vi "PM100D_SetRngIndex.vi"(1 "PM16":bool, 5 "VISAin":refnum<visa-resource-name>, 7 "Unit":string, 9 "AUTO":bool, 11 "error in":errorcluster, 12 "SensType":i32, 13 "Rng_Array":string[](array[string]), 14 "Index":i32) -> (4 "VISAout":refnum<visa-resource-name>, 6 "lblRange":string, 8 "Numeric 2":dbl, 10 "AUTO?":bool, 15 "error out 2":errorcluster)   [LabVIEW 2011]
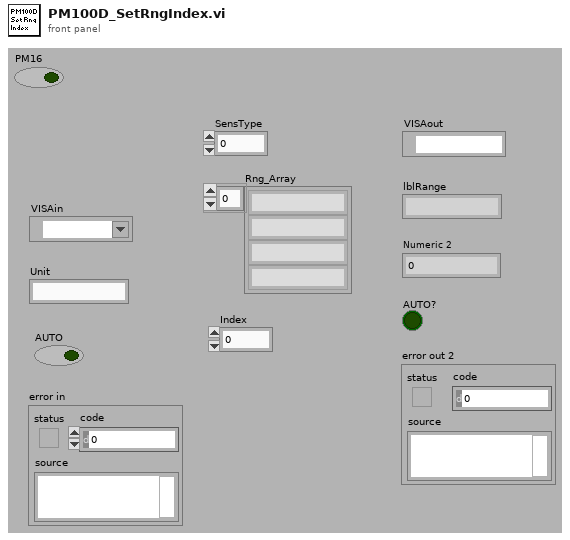
[diagram p1: front panel]
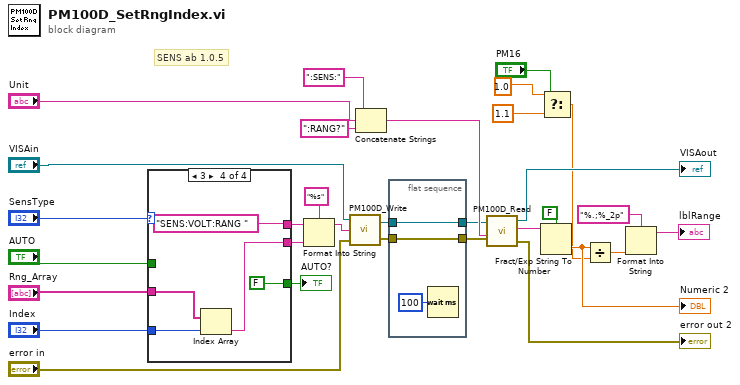
[diagram p0: block diagram]
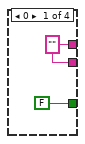
[diagram p2: hidden frame]
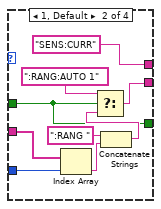
[diagram p3: hidden frame]
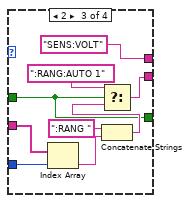
[diagram p4: hidden frame]
diagram:
  # "SENS ab 1.0.5"
  n1 = case shown="3" "SensType" {
    tunnel: [w33 "SENS:CURR" "SENS:VOLT" "SENS:VOLT:RANG " ("string")] -> w18
    tunnel: "Index" -> [_ w42 w51 w56]
    tunnel: "AUTO" -> [_ w34 w43 _]
    tunnel: [w33 w40 w49 w55] -> w20
    tunnel: "Rng_Array" -> [_ w39 w48 w54]
    tunnel: [FALSE ("AUTO") w34 w43 FALSE ("AUTO")] -> w28
    frame 0 {
      w33 = ""
    }
    frame 1, Default {
      n2 = Index Array(array=w39, index=w42) -> (element=w38:string)
      n3 = Concatenate Strings(":RANG " ("string"), w38) -> (w36:string)
      n4 = Select(t=":RANG:AUTO 1", s=w34, f=w36) -> (s? t:f=w40:string)
    }
    frame 2 {
      n5 = Index Array(array=w48, index=w51) -> (element=w45:string)
      n6 = Concatenate Strings(":RANG " ("string"), w45) -> (w44:string)
      n7 = Select(t=":RANG:AUTO 1", s=w43, f=w44) -> (s? t:f=w49:string)
    }
    frame 3 {
      n8 = Index Array(array=w54, index=w56) -> (element=w55:string)
    }
  }
  "AUTO?" <- w28
  n9 = Format Into String(format string="%s", initial string=w18, w20) -> (resulting string=w17:string)  [unwired: 1 in, 1 out]
  n10 = call "PM100D_Write.vi"("error in (no error)"="error in", "Command"=w17, "VISA in"="VISAin") -> ("error out"=w6:errorcluster, "VISA out"=w8:refnum<visa-resource-name>)
  n11 = Concatenate Strings(":SENS:" ("string"), "Unit", ":RANG?" ("string")) -> (w21:string)
  n12 = flat-sequence {
    tunnel: [w59] -> w7
    tunnel: w8 -> [w59]
    tunnel: w6 -> [w58]
    tunnel: [w58] -> w5
    frame #0 {
      n13 = Wait (ms)(milliseconds to wait=u32 100) -> ()  [unwired: 1 out]
    }
  }
  n14 = call "PM100D_Read.vi"("error in (no error)"=w5, "Command"=w21, "VISA in"=w7) -> ("error out"=→"error out 2":errorcluster, "ReadValue"=w12:string, "VISA out"=→"VISAout":refnum<visa-resource-name>)  [unwired: 1 in]
  n15 = Fract/Exp String To Number(use system decimal point (T)=FALSE, string=w12) -> (number=w14:dbl)  [unwired: 2 in, 1 out]
  "Numeric 2" <- w14
  n16 = Select(t=1.0 ("y"), s="PM16", f=1.1) -> (s? t:f=w3:dbl)
  n17 = Divide(x=w14, y=w3) -> (x/y=w15:dbl)
  n18 = Format Into String(format string="%.;%_2p", w15) -> (resulting string=→"lblRange":string)  [unwired: 2 in, 1 out]
